vi "Calculate Number Available (u).vi"(11 "Flag Array":bool[][](array[boolean])) -> (2 "u":i32, 3 "Flag Array Out":bool[][](array[boolean]))   [LabVIEW 2013]
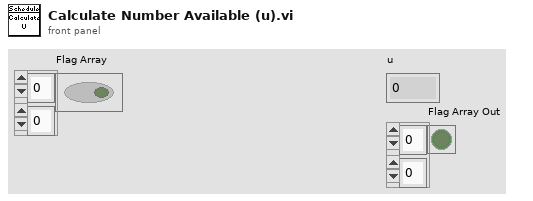
[diagram p1: front panel]
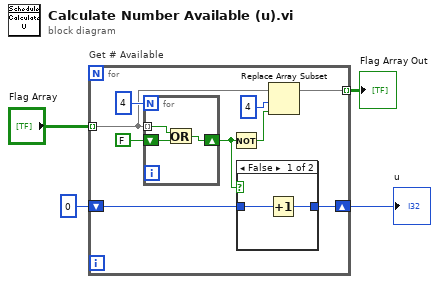
[diagram p0: block diagram]
diagram:
  n1 = for "Get # Available" {
    tunnel: "Flag Array" -> [w8] mode=indexing
    shift-right: [w12] -> w3
    shift-left: 0 -> [w13]
    tunnel: [w5] -> w1 mode=indexing
    n2 = for {
      N: 4 -> [_]
      shift-right: [w14] -> w7
      shift-left: FALSE -> [w15]
      tunnel: w8 -> [w16] mode=indexing
      n3 = Or(x=w16, y=w15) -> (x .or. y?=w14:bool)
    }
    n4 = Not(x=w7) -> (.not. x?=w6:bool)
    n5 = case shown="False" w7 {
      tunnel: w13 -> [w18 w19]
      tunnel: [w17 w19] -> w12
      frame False {
        n6 = Increment(x=w18) -> (x+1=w17:i32)
      }
      frame True {
      }
    }
    n7 = Replace Array Subset(array=w8, new element=w6, index=4) -> (w5:bool[])
  }
  "u" <- w3
  "Flag Array Out" <- w1
